vi "编辑配方.vi"() -> ()   [LabVIEW 2018]
panel:
  in  "退出":bool
  in  "确定写入":bool
  out "说明":string="说明"
  out "详细位置":string="详细位置"
  out "配方编号":string="配方编号"
  out "编辑配方":string[][](array[string])
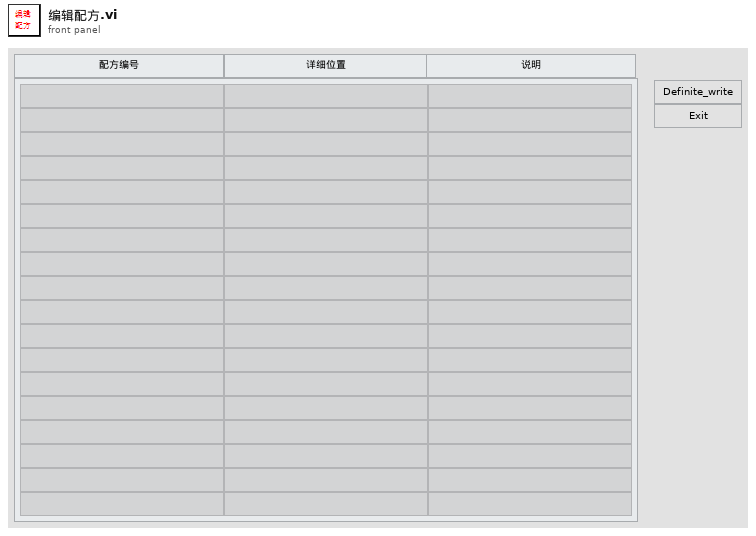
[diagram p1: front panel]
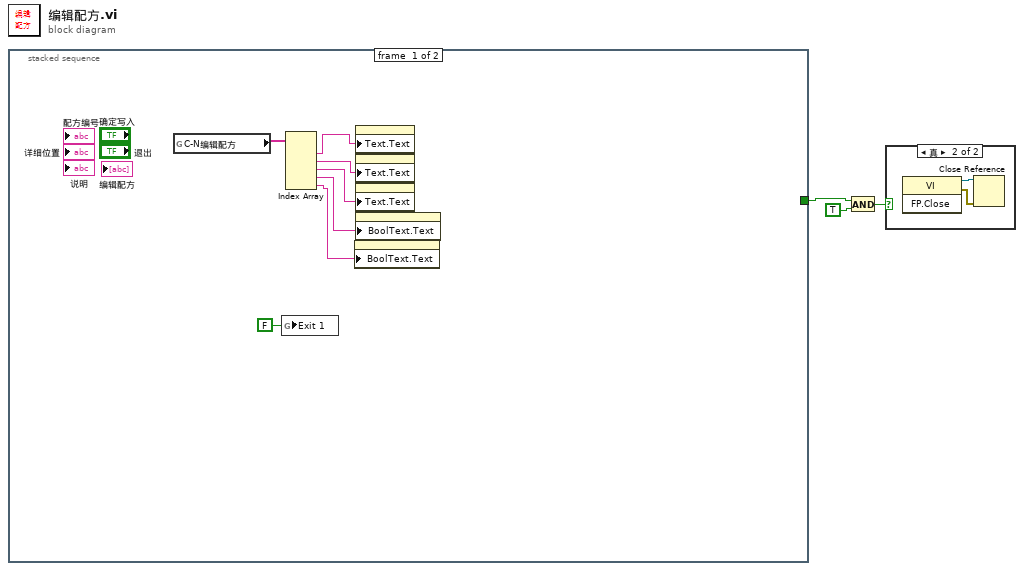
[diagram p0: block diagram]
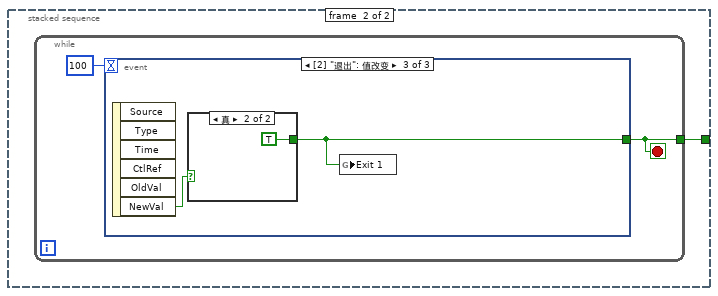
[diagram p2: hidden frame]
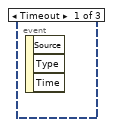
[diagram p3: hidden frame]
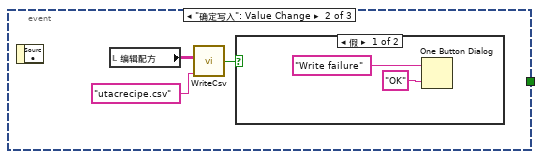
[diagram p4: hidden frame]
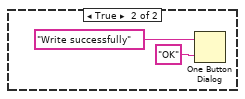
[diagram p5: hidden frame]
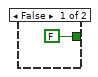
[diagram p6: hidden frame]
diagram:
  n1 = stacked-sequence {
    tunnel: [_ w11] -> w1
    frame #0 {
      n2 = global read "全局 1.vi" "C-N编辑配方"() -> (w10:string[])
      n3 = global write "全局 1.vi" "Exit 1"(FALSE ("Exit 1")) -> ()
      n4 = Index Array(array=w10) -> (element #1=w9:string, element #2=w8:string, element #3=w7:string, element #4=w6:string, element #5=w5:string)  [unwired: 5 in]
      n5 = property on="退出" class="Bool"("BoolText.Text"=w5) -> ()  [unwired: 2 in, 2 out]
      n6 = property on="配方编号" class="Str"("Text.Text"=w9) -> ()  [unwired: 2 in, 2 out]
      n7 = property on="详细位置" class="Str"("Text.Text"=w8) -> ()  [unwired: 2 in, 2 out]
      n8 = property on="说明" class="Str"("Text.Text"=w7) -> ()  [unwired: 2 in, 2 out]
      n9 = property on="确定写入" class="Bool"("BoolText.Text"=w6) -> ()  [unwired: 2 in, 2 out]
    }
    frame #1 {
      n10 = while {
        tunnel: [w12] -> w11
        stop <- w12 stop-if-true
        n11 = event shown="[2] \"退出\": 值改变" {
          selector: _ -> [_ _ _]
          dyn-events: _ -> [_ _ _]
          timeout: 100 -> [_ _ _]
          tunnel: [_ _ w21] -> w12
          event Timeout {
            n12 = event-data() -> ()  [unwired: 1 in, 3 out]
          }
          event "确定写入": Value Change {
            n13 = event-data() -> ()  [unwired: 1 in, 1 out]
            n14 = local read "编辑配方"() -> (w15:string[][])
            n15 = call "WriteCsv.vi"("相对路径"="utacrecipe.csv", "2D data"=w15) -> ("布尔"=w14:bool)  [unwired: 2 in]
            n16 = case shown="假" w14 {
              frame False {
                n17 = One Button Dialog(message="Write failure" ("消息"), button name ("OK")="OK" ("按钮名称（“确定”）")) -> ()  [unwired: 1 out]
              }
              frame True {
                n18 = One Button Dialog(message="Write successfully" ("消息"), button name ("OK")="OK" ("按钮名称（“确定”）")) -> ()  [unwired: 1 out]
              }
            }
          }
          event "退出": Value Change {
            n19 = event-data() -> ("NewVal"=w22:bool)  [unwired: 1 in, 5 out]
            n20 = case shown="真" w22 {
              tunnel: [FALSE TRUE] -> w21
              frame False {
              }
              frame True {
              }
            }
            n21 = global write "全局 1.vi" "Exit 1"(w21) -> ()
          }
        }
      }
    }
  }
  n22 = And(x=w1, y=TRUE) -> (x .and. y?=w2:bool)
  n23 = case shown="真" w2 {
    frame False {
    }
    frame True {
      n24 = invoke class="VI" method="FP.Close"() -> (reference out=w26:refnum<vi>, error out=w25:errorcluster)  [unwired: 3 in, 1 out]
      n25 = Close Reference(reference=w26, error in (no error)=w25) -> ()  [unwired: 1 out]
    }
  }
